vi "Get Class Name and Path.vi"(11 "Class":refnum<class>) -> (1 "Success?":bool, 2 "Class Path":path, 3 "Class Name":string)   [LabVIEW 2020, in "ClassLoader.lvlib"]
doc: "Get base class name (file name without extension) and path to the given class."
uses:
  ClassLoader.lvlib
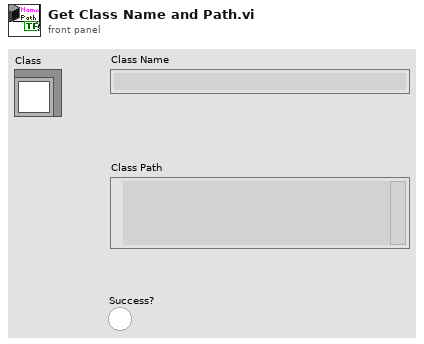
[diagram p1: front panel]
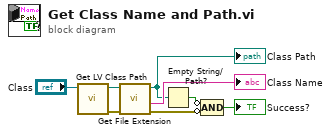
[diagram p0: block diagram]
diagram:
  n1 = call <vilib>:"Get LV Class Path.vi"("object"="Class") -> ("error out"=w7:errorcluster, "class path"=w6:path)  [unwired: 9 in]
  n2 = call <vilib>:"Get File Extension.vi"("error in (no error)"=w7, "file"=w6) -> ("error out"=w2:errorcluster, "filename without extension"=→"Class Name":string, "dup file"=w4:path)  [unwired: 5 in, 2 out]
  "Class Path" <- w4
  n3 = Empty String/Path?(string/path=w4) -> (empty?=w3:bool)
  n4 = Compound Arithmetic op=AND(invert w3, invert w2) -> (→"Success?":bool)
